vi "Lab Panel V5.31.vi"() -> ()   [LabVIEW 2017] (continued)
                n1120 = Equal?(x=w2128, y="RUN") -> (x = y?=w2130:bool)
                n1121 = And(x=w2130, y=w2131) -> (x .and. y?=w2129:bool)
                n1122 = case shown="True" w2129 {
                  tunnel: w2134 -> [_ w2139]
                  tunnel: w2133 -> [_ w2143]
                  frame False {
                  }
                  frame True {
                    n1123 = local read "SET LAB01-1"() -> (w2145:T6)
                    n1124 = local read "TDMS LAB01-1"() -> (w2138:refnum<k34>)
                    n1125 = Unbundle(w2145) -> ("CYCLES"=w2136:dbl, "T-RISE mins"=w2142:dbl)  [unwired: 3 out]
                    n1126 = case shown="\"CYCLE TEST\"" w2143 {
                      tunnel: w2142 -> [_ _ w2152]
                      tunnel: [w2147 w2149 w2152] -> w2141
                      tunnel: w2136 -> [w2147 w2149 _]
                      tunnel: ["CHART PASS" "CYCLE PASS" "T-RISE PASS"] -> w2140
                      frame "CHART TEST", Default {
                      }
                      frame "CYCLE TEST" {
                      }
                      frame "T-RISE TEST" {
                      }
                    }
                    n1127 = Unbundle(w2139) -> ("CYCLE"=w2144:dbl)  [unwired: 2 out]
                    n1128 = Increment(x=w2136) -> (x+1=w2137:dbl)
                    n1129 = Greater Or Equal?(x=w2144, y=w2137) -> (x >= y?=w2146:bool)
                    n1130 = case shown="True" w2146 {
                      tunnel: w2141 -> [w2156 _]
                      tunnel: w2140 -> [w2155 _]
                      tunnel: w2139 -> [w2154 _]
                      tunnel: w2138 -> [w2153 _]
                      frame True {
                        n1131 = stacked-sequence {
                          tunnel: w2156 -> [w2160 _]
                          tunnel: w2155 -> [w2158 w2164]
                          tunnel: w2154 -> [_ w2167]
                          tunnel: w2153 -> [w2157 _]
                          frame #0 {
                            n1132 = Build Array(w2158) -> (w2161:string[])
                            n1133 = Build Array(w2160) -> (w2159:dbl[])
                            n1134 = TDMS Write(0:w2157, 5:"TEST PASS", 7:w2161, 9:w2159) -> (15:w2163:errorcluster)  [unwired: 2 in, 3 out]
                            n1135 = local write "data file error"(w2163) -> ()
                          }
                          frame #1 {
                            n1136 = Bundle(cluster=w2167, "STATUS"=w2164) -> (w2165:T4)  [unwired: 2 in]
                            n1137 = local write "RESULT LAB01-1"(TRUE) -> ()
                            n1138 = local write "DISP LAB01-1"(w2165) -> ()
                          }
                        }
                      }
                      frame False {
                      }
                    }
                  }
                }
              }
              frame #1 {
                # "LAB01-2"
                n1139 = Less?(x=w2168, y=2) -> (x < y?=w2171:bool)
                n1140 = local read "DISP LAB01-2"() -> (w2173:T4)
                n1141 = Unbundle(w2173) -> ("STATUS"=w2174:string)  [unwired: 2 out]
                n1142 = Equal?(x=w2174, y="RUN") -> (x = y?=w2170:bool)
                n1143 = And(x=w2170, y=w2171) -> (x .and. y?=w2169:bool)
                n1144 = case shown="True" w2169 {
                  tunnel: w2173 -> [_ w2179]
                  tunnel: w2168 -> [_ w2183]
                  frame False {
                  }
                  frame True {
                    n1145 = local read "SET LAB01-2"() -> (w2185:T5)
                    n1146 = local read "TDMS LAB01-2"() -> (w2178:refnum<k34>)
                    n1147 = Unbundle(w2185) -> ("CYCLES"=w2176:dbl, "T-RISE mins"=w2182:dbl)  [unwired: 3 out]
                    n1148 = case shown="\"T-RISE TEST\"" w2183 {
                      tunnel: w2182 -> [_ _ w2192]
                      tunnel: [w2187 w2189 w2192] -> w2181
                      tunnel: w2176 -> [w2187 w2189 _]
                      tunnel: ["CHART PASS" "CYCLE PASS" "T-RISE PASS"] -> w2180
                      frame "CHART TEST", Default {
                      }
                      frame "CYCLE TEST" {
                      }
                      frame "T-RISE TEST" {
                      }
                    }
                    n1149 = Unbundle(w2179) -> ("CYCLE"=w2184:dbl)  [unwired: 2 out]
                    n1150 = Increment(x=w2176) -> (x+1=w2177:dbl)
                    n1151 = Greater Or Equal?(x=w2184, y=w2177) -> (x >= y?=w2186:bool)
                    n1152 = case shown="True" w2186 {
                      tunnel: w2181 -> [w2196 _]
                      tunnel: w2180 -> [w2195 _]
                      tunnel: w2179 -> [w2194 _]
                      tunnel: w2178 -> [w2193 _]
                      frame True {
                        n1153 = stacked-sequence {
                          tunnel: w2196 -> [w2200 _]
                          tunnel: w2195 -> [w2198 w2204]
                          tunnel: w2194 -> [_ w2207]
                          tunnel: w2193 -> [w2197 _]
                          frame #0 {
                            n1154 = Build Array(w2198) -> (w2201:string[])
                            n1155 = Build Array(w2200) -> (w2199:dbl[])
                            n1156 = TDMS Write(0:w2197, 5:"TEST PASS", 7:w2201, 9:w2199) -> (15:w2203:errorcluster)  [unwired: 2 in, 3 out]
                            n1157 = local write "data file error"(w2203) -> ()
                          }
                          frame #1 {
                            n1158 = Bundle(cluster=w2207, "STATUS"=w2204) -> (w2205:T4)  [unwired: 2 in]
                            n1159 = local write "RESULT LAB01-2"(TRUE) -> ()
                            n1160 = local write "DISP LAB01-2"(w2205) -> ()
                          }
                        }
                      }
                      frame False {
                      }
                    }
                  }
                }
              }
              frame #2 {
                # "LAB02-1"
                n1161 = Less?(x=w2208, y=2) -> (x < y?=w2211:bool)
                n1162 = local read "DISP LAB02-1"() -> (w2213:T4)
                n1163 = Unbundle(w2213) -> ("STATUS"=w2214:string)  [unwired: 2 out]
                n1164 = Equal?(x=w2214, y="RUN") -> (x = y?=w2210:bool)
                n1165 = And(x=w2210, y=w2211) -> (x .and. y?=w2209:bool)
                n1166 = case shown="True" w2209 {
                  tunnel: w2213 -> [_ w2219]
                  tunnel: w2208 -> [_ w2223]
                  frame False {
                  }
                  frame True {
                    n1167 = local read "TDMS LAB02-1"() -> (w2218:refnum<k34>)
                    n1168 = local read "SET LAB02-1"() -> (w2225:T5)
                    n1169 = Unbundle(w2219) -> ("CYCLE"=w2224:dbl)  [unwired: 2 out]
                    n1170 = Unbundle(w2225) -> ("CYCLES"=w2216:dbl, "T-RISE mins"=w2222:dbl)  [unwired: 3 out]
                    n1171 = case shown="\"T-RISE TEST\"" w2223 {
                      tunnel: w2222 -> [_ _ w2232]
                      tunnel: [w2227 w2229 w2232] -> w2221
                      tunnel: w2216 -> [w2227 w2229 _]
                      tunnel: ["CHART PASS" "CYCLE PASS" "T-RISE PASS"] -> w2220
                      frame "CHART TEST", Default {
                      }
                      frame "CYCLE TEST" {
                      }
                      frame "T-RISE TEST" {
                      }
                    }
                    n1172 = Increment(x=w2216) -> (x+1=w2217:dbl)
                    n1173 = Greater Or Equal?(x=w2224, y=w2217) -> (x >= y?=w2226:bool)
                    n1174 = case shown="True" w2226 {
                      tunnel: w2221 -> [w2236 _]
                      tunnel: w2220 -> [w2235 _]
                      tunnel: w2219 -> [w2234 _]
                      tunnel: w2218 -> [w2233 _]
                      frame True {
                        n1175 = stacked-sequence {
                          tunnel: w2236 -> [w2240 _]
                          tunnel: w2235 -> [w2238 w2244]
                          tunnel: w2234 -> [_ w2247]
                          tunnel: w2233 -> [w2237 _]
                          frame #0 {
                            n1176 = Build Array(w2238) -> (w2241:string[])
                            n1177 = Build Array(w2240) -> (w2239:dbl[])
                            n1178 = TDMS Write(0:w2237, 5:"TEST PASS", 7:w2241, 9:w2239) -> (15:w2243:errorcluster)  [unwired: 2 in, 3 out]
                            n1179 = local write "data file error"(w2243) -> ()
                          }
                          frame #1 {
                            n1180 = Bundle(cluster=w2247, "STATUS"=w2244) -> (w2245:T4)  [unwired: 2 in]
                            n1181 = local write "RESULT LAB02-1"(TRUE) -> ()
                            n1182 = local write "DISP LAB02-1"(w2245) -> ()
                          }
                        }
                      }
                      frame False {
                      }
                    }
                  }
                }
              }
              frame #3 {
                # "LAB02-2"
                n1183 = Less?(x=w2248, y=2) -> (x < y?=w2251:bool)
                n1184 = local read "DISP LAB02-2"() -> (w2253:T4)
                n1185 = Unbundle(w2253) -> ("STATUS"=w2254:string)  [unwired: 2 out]
                n1186 = Equal?(x=w2254, y="RUN") -> (x = y?=w2250:bool)
                n1187 = And(x=w2250, y=w2251) -> (x .and. y?=w2249:bool)
                n1188 = case shown="True" w2249 {
                  tunnel: w2253 -> [_ w2259]
                  tunnel: w2248 -> [_ w2263]
                  frame False {
                  }
                  frame True {
                    n1189 = local read "TDMS LAB02-2"() -> (w2258:refnum<k34>)
                    n1190 = local read "SET LAB02-2"() -> (w2265:T5)
                    n1191 = Unbundle(w2259) -> ("CYCLE"=w2264:dbl)  [unwired: 2 out]
                    n1192 = Unbundle(w2265) -> ("CYCLES"=w2256:dbl, "T-RISE mins"=w2262:dbl)  [unwired: 3 out]
                    n1193 = case shown="\"T-RISE TEST\"" w2263 {
                      tunnel: w2262 -> [_ _ w2272]
                      tunnel: [w2267 w2269 w2272] -> w2261
                      tunnel: w2256 -> [w2267 w2269 _]
                      tunnel: ["CHART PASS" "CYCLE PASS" "T-RISE PASS"] -> w2260
                      frame "CHART TEST", Default {
                      }
                      frame "CYCLE TEST" {
                      }
                      frame "T-RISE TEST" {
                      }
                    }
                    n1194 = Increment(x=w2256) -> (x+1=w2257:dbl)
                    n1195 = Greater Or Equal?(x=w2264, y=w2257) -> (x >= y?=w2266:bool)
                    n1196 = case shown="True" w2266 {
                      tunnel: w2261 -> [w2276 _]
                      tunnel: w2260 -> [w2275 _]
                      tunnel: w2259 -> [w2274 _]
                      tunnel: w2258 -> [w2273 _]
                      frame True {
                        n1197 = stacked-sequence {
                          tunnel: w2276 -> [w2280 _]
                          tunnel: w2275 -> [w2278 w2284]
                          tunnel: w2274 -> [_ w2287]
                          tunnel: w2273 -> [w2277 _]
                          frame #0 {
                            n1198 = Build Array(w2278) -> (w2281:string[])
                            n1199 = Build Array(w2280) -> (w2279:dbl[])
                            n1200 = TDMS Write(0:w2277, 5:"TEST PASS", 7:w2281, 9:w2279) -> (15:w2283:errorcluster)  [unwired: 2 in, 3 out]
                            n1201 = local write "data file error"(w2283) -> ()
                          }
                          frame #1 {
                            n1202 = Bundle(cluster=w2287, "STATUS"=w2284) -> (w2285:T4)  [unwired: 2 in]
                            n1203 = local write "RESULT LAB02-2"(TRUE) -> ()
                            n1204 = local write "DISP LAB02-2"(w2285) -> ()
                          }
                        }
                      }
                      frame False {
                      }
                    }
                  }
                }
              }
              frame #4 {
                # "LAB03-1"
                n1205 = Less?(x=w2288, y=2) -> (x < y?=w2291:bool)
                n1206 = local read "DISP LAB03-1"() -> (w2293:T4)
                n1207 = Unbundle(w2293) -> ("STATUS"=w2294:string)  [unwired: 2 out]
                n1208 = Equal?(x=w2294, y="RUN") -> (x = y?=w2290:bool)
                n1209 = And(x=w2290, y=w2291) -> (x .and. y?=w2289:bool)
                n1210 = case shown="True" w2289 {
                  tunnel: w2293 -> [_ w2299]
                  tunnel: w2288 -> [_ w2303]
                  frame False {
                  }
                  frame True {
                    n1211 = local read "TDMS LAB03-1"() -> (w2298:refnum<k34>)
                    n1212 = local read "SET LAB03-1"() -> (w2305:T5)
                    n1213 = Unbundle(w2299) -> ("CYCLE"=w2304:dbl)  [unwired: 2 out]
                    n1214 = Unbundle(w2305) -> ("CYCLES"=w2296:dbl, "T-RISE mins"=w2302:dbl)  [unwired: 3 out]
                    n1215 = case shown="\"T-RISE TEST\"" w2303 {
                      tunnel: w2302 -> [_ _ w2312]
                      tunnel: [w2307 w2309 w2312] -> w2301
                      tunnel: w2296 -> [w2307 w2309 _]
                      tunnel: ["CHART PASS" "CYCLE PASS" "T-RISE PASS"] -> w2300
                      frame "CHART TEST", Default {
                      }
                      frame "CYCLE TEST" {
                      }
                      frame "T-RISE TEST" {
                      }
                    }
                    n1216 = Increment(x=w2296) -> (x+1=w2297:dbl)
                    n1217 = Greater Or Equal?(x=w2304, y=w2297) -> (x >= y?=w2306:bool)
                    n1218 = case shown="True" w2306 {
                      tunnel: w2301 -> [w2316 _]
                      tunnel: w2300 -> [w2315 _]
                      tunnel: w2299 -> [w2314 _]
                      tunnel: w2298 -> [w2313 _]
                      frame True {
                        n1219 = stacked-sequence {
                          tunnel: w2316 -> [w2320 _]
                          tunnel: w2315 -> [w2318 w2324]
                          tunnel: w2314 -> [_ w2327]
                          tunnel: w2313 -> [w2317 _]
                          frame #0 {
                            n1220 = Build Array(w2318) -> (w2321:string[])
                            n1221 = Build Array(w2320) -> (w2319:dbl[])
                            n1222 = TDMS Write(0:w2317, 5:"TEST PASS", 7:w2321, 9:w2319) -> (15:w2323:errorcluster)  [unwired: 2 in, 3 out]
                            n1223 = local write "data file error"(w2323) -> ()
                          }
                          frame #1 {
                            n1224 = Bundle(cluster=w2327, "STATUS"=w2324) -> (w2325:T4)  [unwired: 2 in]
                            n1225 = local write "RESULT LAB03-1"(TRUE) -> ()
                            n1226 = local write "DISP LAB03-1"(w2325) -> ()
                          }
                        }
                      }
                      frame False {
                      }
                    }
                  }
                }
              }
              frame #5 {
                # "LAB03-2"
                n1227 = Less?(x=w2328, y=2) -> (x < y?=w2331:bool)
                n1228 = local read "DISP LAB03-2"() -> (w2333:T4)
                n1229 = Unbundle(w2333) -> ("STATUS"=w2334:string)  [unwired: 2 out]
                n1230 = Equal?(x=w2334, y="RUN") -> (x = y?=w2330:bool)
                n1231 = And(x=w2330, y=w2331) -> (x .and. y?=w2329:bool)
                n1232 = case shown="True" w2329 {
                  tunnel: w2333 -> [_ w2339]
                  tunnel: w2328 -> [_ w2343]
                  frame False {
                  }
                  frame True {
                    n1233 = local read "TDMS LAB03-2"() -> (w2338:refnum<k34>)
                    n1234 = local read "SET LAB03-2"() -> (w2345:T5)
                    n1235 = Unbundle(w2339) -> ("CYCLE"=w2344:dbl)  [unwired: 2 out]
                    n1236 = Unbundle(w2345) -> ("CYCLES"=w2336:dbl, "T-RISE mins"=w2342:dbl)  [unwired: 3 out]
                    n1237 = case shown="\"T-RISE TEST\"" w2343 {
                      tunnel: w2342 -> [_ _ w2352]
                      tunnel: [w2347 w2349 w2352] -> w2341
                      tunnel: w2336 -> [w2347 w2349 _]
                      tunnel: ["CHART PASS" "CYCLE PASS" "T-RISE PASS"] -> w2340
                      frame "CHART TEST", Default {
                      }
                      frame "CYCLE TEST" {
                      }
                      frame "T-RISE TEST" {
                      }
                    }
                    n1238 = Increment(x=w2336) -> (x+1=w2337:dbl)
                    n1239 = Greater Or Equal?(x=w2344, y=w2337) -> (x >= y?=w2346:bool)
                    n1240 = case shown="True" w2346 {
                      tunnel: w2341 -> [w2356 _]
                      tunnel: w2340 -> [w2355 _]
                      tunnel: w2339 -> [w2354 _]
                      tunnel: w2338 -> [w2353 _]
                      frame True {
                        n1241 = stacked-sequence {
                          tunnel: w2356 -> [w2360 _]
                          tunnel: w2355 -> [w2358 w2364]
                          tunnel: w2354 -> [_ w2367]
                          tunnel: w2353 -> [w2357 _]
                          frame #0 {
                            n1242 = Build Array(w2358) -> (w2361:string[])
                            n1243 = Build Array(w2360) -> (w2359:dbl[])
                            n1244 = TDMS Write(0:w2357, 5:"TEST PASS", 7:w2361, 9:w2359) -> (15:w2363:errorcluster)  [unwired: 2 in, 3 out]
                            n1245 = local write "data file error"(w2363) -> ()
                          }
                          frame #1 {
                            n1246 = Bundle(cluster=w2367, "STATUS"=w2364) -> (w2365:T4)  [unwired: 2 in]
                            n1247 = local write "RESULT LAB03-2"(TRUE) -> ()
                            n1248 = local write "DISP LAB03-2"(w2365) -> ()
                          }
                        }
                      }
                      frame False {
                      }
                    }
                  }
                }
              }
              frame #6 {
                # "LAB04-1"
                n1249 = Less?(x=w2368, y=2) -> (x < y?=w2371:bool)
                n1250 = local read "DISP LAB04-1"() -> (w2373:T4)
                n1251 = Unbundle(w2373) -> ("STATUS"=w2374:string)  [unwired: 2 out]
                n1252 = Equal?(x=w2374, y="RUN") -> (x = y?=w2370:bool)
                n1253 = And(x=w2370, y=w2371) -> (x .and. y?=w2369:bool)
                n1254 = case shown="True" w2369 {
                  tunnel: w2373 -> [_ w2379]
                  tunnel: w2368 -> [_ w2383]
                  frame False {
                  }
                  frame True {
                    n1255 = local read "TDMS LAB04-1"() -> (w2378:refnum<k34>)
                    n1256 = local read "SET LAB04-1"() -> (w2385:T5)
                    n1257 = Unbundle(w2379) -> ("CYCLE"=w2384:dbl)  [unwired: 2 out]
                    n1258 = Unbundle(w2385) -> ("CYCLES"=w2376:dbl, "T-RISE mins"=w2382:dbl)  [unwired: 3 out]
                    n1259 = case shown="\"T-RISE TEST\"" w2383 {
                      tunnel: w2382 -> [_ _ w2392]
                      tunnel: [w2387 w2389 w2392] -> w2381
                      tunnel: w2376 -> [w2387 w2389 _]
                      tunnel: ["CHART PASS" "CYCLE PASS" "T-RISE PASS"] -> w2380
                      frame "CHART TEST", Default {
                      }
                      frame "CYCLE TEST" {
                      }
                      frame "T-RISE TEST" {
                      }
                    }
                    n1260 = Increment(x=w2376) -> (x+1=w2377:dbl)
                    n1261 = Greater Or Equal?(x=w2384, y=w2377) -> (x >= y?=w2386:bool)
                    n1262 = case shown="True" w2386 {
                      tunnel: w2381 -> [w2396 _]
                      tunnel: w2380 -> [w2395 _]
                      tunnel: w2379 -> [w2394 _]
                      tunnel: w2378 -> [w2393 _]
                      frame True {
                        n1263 = stacked-sequence {
                          tunnel: w2396 -> [w2400 _]
                          tunnel: w2395 -> [w2398 w2404]
                          tunnel: w2394 -> [_ w2407]
                          tunnel: w2393 -> [w2397 _]
                          frame #0 {
                            n1264 = Build Array(w2398) -> (w2401:string[])
                            n1265 = Build Array(w2400) -> (w2399:dbl[])
                            n1266 = TDMS Write(0:w2397, 5:"TEST PASS", 7:w2401, 9:w2399) -> (15:w2403:errorcluster)  [unwired: 2 in, 3 out]
                            n1267 = local write "data file error"(w2403) -> ()
                          }
                          frame #1 {
                            n1268 = Bundle(cluster=w2407, "STATUS"=w2404) -> (w2405:T4)  [unwired: 2 in]
                            n1269 = local write "RESULT LAB04-1"(TRUE) -> ()
                            n1270 = local write "DISP LAB04-1"(w2405) -> ()
                          }
                        }
                      }
                      frame False {
                      }
                    }
                  }
                }
              }
              frame #7 {
                # "LAB04-2"
                n1271 = Less?(x=w2408, y=2) -> (x < y?=w2411:bool)
                n1272 = local read "DISP LAB04-2"() -> (w2413:T4)
                n1273 = Unbundle(w2413) -> ("STATUS"=w2414:string)  [unwired: 2 out]
                n1274 = Equal?(x=w2414, y="RUN") -> (x = y?=w2410:bool)
                n1275 = And(x=w2410, y=w2411) -> (x .and. y?=w2409:bool)
                n1276 = case shown="True" w2409 {
                  tunnel: w2413 -> [_ w2419]
                  tunnel: w2408 -> [_ w2423]
                  frame False {
                  }
                  frame True {
                    n1277 = local read "TDMS LAB04-2"() -> (w2418:refnum<k34>)
                    n1278 = local read "SET LAB04-2"() -> (w2425:T5)
                    n1279 = Unbundle(w2419) -> ("CYCLE"=w2424:dbl)  [unwired: 2 out]
                    n1280 = Unbundle(w2425) -> ("CYCLES"=w2416:dbl, "T-RISE mins"=w2422:dbl)  [unwired: 3 out]
                    n1281 = case shown="\"T-RISE TEST\"" w2423 {
                      tunnel: w2422 -> [_ _ w2432]
                      tunnel: [w2427 w2429 w2432] -> w2421
                      tunnel: w2416 -> [w2427 w2429 _]
                      tunnel: ["CHART PASS" "CYCLE PASS" "T-RISE PASS"] -> w2420
                      frame "CHART TEST", Default {
                      }
                      frame "CYCLE TEST" {
                      }
                      frame "T-RISE TEST" {
                      }
                    }
                    n1282 = Increment(x=w2416) -> (x+1=w2417:dbl)
                    n1283 = Greater Or Equal?(x=w2424, y=w2417) -> (x >= y?=w2426:bool)
                    n1284 = case shown="True" w2426 {
                      tunnel: w2421 -> [w2436 _]
                      tunnel: w2420 -> [w2435 _]
                      tunnel: w2419 -> [w2434 _]
                      tunnel: w2418 -> [w2433 _]
                      frame True {
                        n1285 = stacked-sequence {
                          tunnel: w2436 -> [w2440 _]
                          tunnel: w2435 -> [w2438 w2444]
                          tunnel: w2434 -> [_ w2447]
                          tunnel: w2433 -> [w2437 _]
                          frame #0 {
                            n1286 = Build Array(w2438) -> (w2441:string[])
                            n1287 = Build Array(w2440) -> (w2439:dbl[])
                            n1288 = TDMS Write(0:w2437, 5:"TEST PASS", 7:w2441, 9:w2439) -> (15:w2443:errorcluster)  [unwired: 2 in, 3 out]
                            n1289 = local write "data file error"(w2443) -> ()
                          }
                          frame #1 {
                            n1290 = Bundle(cluster=w2447, "STATUS"=w2444) -> (w2445:T4)  [unwired: 2 in]
                            n1291 = local write "RESULT LAB04-2"(TRUE) -> ()
                            n1292 = local write "DISP LAB04-2"(w2445) -> ()
                          }
                        }
                      }
                      frame False {
                      }
                    }
                  }
                }
              }
              frame #8 {
                # "LAB05-1"
                n1293 = Less?(x=w2448, y=2) -> (x < y?=w2451:bool)
                n1294 = local read "DISP LAB05-1"() -> (w2453:T4)
                n1295 = Unbundle(w2453) -> ("STATUS"=w2454:string)  [unwired: 2 out]
                n1296 = Equal?(x=w2454, y="RUN") -> (x = y?=w2450:bool)
                n1297 = And(x=w2450, y=w2451) -> (x .and. y?=w2449:bool)
                n1298 = case shown="True" w2449 {
                  tunnel: w2453 -> [_ w2459]
                  tunnel: w2448 -> [_ w2463]
                  frame False {
                  }
                  frame True {
                    n1299 = local read "TDMS LAB05-1"() -> (w2458:refnum<k34>)
                    n1300 = local read "SET LAB05-1"() -> (w2465:T5)
                    n1301 = Unbundle(w2459) -> ("CYCLE"=w2464:dbl)  [unwired: 2 out]
                    n1302 = Unbundle(w2465) -> ("CYCLES"=w2456:dbl, "T-RISE mins"=w2462:dbl)  [unwired: 3 out]
                    n1303 = case shown="\"T-RISE TEST\"" w2463 {
                      tunnel: w2462 -> [_ _ w2472]
                      tunnel: [w2467 w2469 w2472] -> w2461
                      tunnel: w2456 -> [w2467 w2469 _]
                      tunnel: ["CHART PASS" "CYCLE PASS" "T-RISE PASS"] -> w2460
                      frame "CHART TEST", Default {
                      }
                      frame "CYCLE TEST" {
                      }
                      frame "T-RISE TEST" {
                      }
                    }
                    n1304 = Increment(x=w2456) -> (x+1=w2457:dbl)
                    n1305 = Greater Or Equal?(x=w2464, y=w2457) -> (x >= y?=w2466:bool)
                    n1306 = case shown="True" w2466 {
                      tunnel: w2461 -> [w2476 _]
                      tunnel: w2460 -> [w2475 _]
                      tunnel: w2459 -> [w2474 _]
                      tunnel: w2458 -> [w2473 _]
                      frame True {
                        n1307 = stacked-sequence {
                          tunnel: w2476 -> [w2480 _]
                          tunnel: w2475 -> [w2478 w2484]
                          tunnel: w2474 -> [_ w2487]
                          tunnel: w2473 -> [w2477 _]
                          frame #0 {
                            n1308 = Build Array(w2478) -> (w2481:string[])
                            n1309 = Build Array(w2480) -> (w2479:dbl[])
                            n1310 = TDMS Write(0:w2477, 5:"TEST PASS", 7:w2481, 9:w2479) -> (15:w2483:errorcluster)  [unwired: 2 in, 3 out]
                            n1311 = local write "data file error"(w2483) -> ()
                          }
                          frame #1 {
                            n1312 = Bundle(cluster=w2487, "STATUS"=w2484) -> (w2485:T4)  [unwired: 2 in]
                            n1313 = local write "RESULT LAB05-1"(TRUE) -> ()
                            n1314 = local write "DISP LAB05-1"(w2485) -> ()
                          }
                        }
                      }
                      frame False {
                      }
                    }
                  }
                }
              }
              frame #9 {
                # "LAB05-2"
                n1315 = Less?(x=w2488, y=2) -> (x < y?=w2491:bool)
                n1316 = local read "DISP LAB05-2"() -> (w2493:T4)
                n1317 = Unbundle(w2493) -> ("STATUS"=w2494:string)  [unwired: 2 out]
                n1318 = Equal?(x=w2494, y="RUN") -> (x = y?=w2490:bool)
                n1319 = And(x=w2490, y=w2491) -> (x .and. y?=w2489:bool)
                n1320 = case shown="True" w2489 {
                  tunnel: w2493 -> [_ w2499]
                  tunnel: w2488 -> [_ w2503]
                  frame False {
                  }
                  frame True {
                    n1321 = local read "TDMS LAB05-2"() -> (w2498:refnum<k34>)
                    n1322 = local read "SET LAB05-2"() -> (w2505:T5)
                    n1323 = Unbundle(w2499) -> ("CYCLE"=w2504:dbl)  [unwired: 2 out]
                    n1324 = Unbundle(w2505) -> ("CYCLES"=w2496:dbl, "T-RISE mins"=w2502:dbl)  [unwired: 3 out]
                    n1325 = case shown="\"T-RISE TEST\"" w2503 {
                      tunnel: w2502 -> [_ _ w2512]
                      tunnel: [w2507 w2509 w2512] -> w2501
                      tunnel: w2496 -> [w2507 w2509 _]
                      tunnel: ["CHART PASS" "CYCLE PASS" "T-RISE PASS"] -> w2500
                      frame "CHART TEST", Default {
                      }
                      frame "CYCLE TEST" {
                      }
                      frame "T-RISE TEST" {
                      }
                    }
                    n1326 = Increment(x=w2496) -> (x+1=w2497:dbl)
                    n1327 = Greater Or Equal?(x=w2504, y=w2497) -> (x >= y?=w2506:bool)
                    n1328 = case shown="True" w2506 {
                      tunnel: w2501 -> [w2516 _]
                      tunnel: w2500 -> [w2515 _]
                      tunnel: w2499 -> [w2514 _]
                      tunnel: w2498 -> [w2513 _]
                      frame True {
                        n1329 = stacked-sequence {
                          tunnel: w2516 -> [w2520 _]
                          tunnel: w2515 -> [w2518 w2524]
                          tunnel: w2514 -> [_ w2527]
                          tunnel: w2513 -> [w2517 _]
                          frame #0 {
                            n1330 = Build Array(w2518) -> (w2521:string[])
                            n1331 = Build Array(w2520) -> (w2519:dbl[])
                            n1332 = TDMS Write(0:w2517, 5:"TEST PASS", 7:w2521, 9:w2519) -> (15:w2523:errorcluster)  [unwired: 2 in, 3 out]
                            n1333 = local write "data file error"(w2523) -> ()
                          }
                          frame #1 {
                            n1334 = Bundle(cluster=w2527, "STATUS"=w2524) -> (w2525:T4)  [unwired: 2 in]
                            n1335 = local write "RESULT LAB05-2"(TRUE) -> ()
                            n1336 = local write "DISP LAB05-2"(w2525) -> ()
                          }
                        }
                      }
                      frame False {
                      }
                    }
                  }
                }
              }
            }
          }
          frame #6 {
            # "check if test cycles reached for temperature rise test"
            n1337 = stacked-sequence {
              tunnel: w2557 -> [_ _ _ _ _ _ _ _ _ _]
              tunnel: w2556 -> [_ _ _ _ _ _ _ _ _ _]
              tunnel: w2555 -> [_ _ _ _ _ _ _ _ _ _]
              tunnel: w2554 -> [_ _ _ _ _ _ _ _ _ _]
              tunnel: w2553 -> [_ _ _ _ _ _ _ _ _ _]
              tunnel: w2552 -> [_ _ _ _ _ _ _ _ _ _]
              tunnel: w2551 -> [_ _ _ _ _ _ _ _ _ _]
              tunnel: w2550 -> [_ _ _ _ _ _ _ _ _ _]
              tunnel: w2549 -> [_ _ _ _ _ _ _ _ _ _]
              tunnel: w2548 -> [_ _ _ _ _ _ _ _ _ _]
              tunnel: w2547 -> [w2563 _ _ _ _ _ _ _ _ _]
              tunnel: w2537 -> [w2558 _ _ _ _ _ _ _ _ _]
              tunnel: w2546 -> [_ w2589 _ _ _ _ _ _ _ _]
              tunnel: w2545 -> [_ _ w2619 _ _ _ _ _ _ _]
              tunnel: w2544 -> [_ _ _ w2649 _ _ _ _ _ _]
              tunnel: w2543 -> [_ _ _ _ w2679 _ _ _ _ _]
              tunnel: w2542 -> [_ _ _ _ _ w2709 _ _ _ _]
              tunnel: w2541 -> [_ _ _ _ _ _ w2739 _ _ _]
              tunnel: w2540 -> [_ _ _ _ _ _ _ w2769 _ _]
              tunnel: w2539 -> [_ _ _ _ _ _ _ _ w2799 _]
              tunnel: w2538 -> [_ _ _ _ _ _ _ _ _ w2829]
              tunnel: w2536 -> [_ w2588 _ _ _ _ _ _ _ _]
              tunnel: w2535 -> [_ _ w2618 _ _ _ _ _ _ _]
              tunnel: w2534 -> [_ _ _ w2648 _ _ _ _ _ _]
              tunnel: w2533 -> [_ _ _ _ w2678 _ _ _ _ _]
              tunnel: w2532 -> [_ _ _ _ _ w2708 _ _ _ _]
              tunnel: w2531 -> [_ _ _ _ _ _ w2738 _ _ _]
              tunnel: w2530 -> [_ _ _ _ _ _ _ w2768 _ _]
              tunnel: w2529 -> [_ _ _ _ _ _ _ _ w2798 _]
              tunnel: w2528 -> [_ _ _ _ _ _ _ _ _ w2828]
              frame #0 {
                # "LAB01-1"
                n1338 = Equal?(x=w2563, y=2) -> (x = y?=w2561:bool)
                n1339 = local read "DISP LAB01-1"() -> (w2564:T4)
                n1340 = Unbundle By Name(w2564) -> ("STATUS"=w2565:string)
                n1341 = Equal?(x=w2565, y="RUN") -> (x = y?=w2560:bool)
                n1342 = And(x=w2560, y=w2561) -> (x .and. y?=w2559:bool)
                n1343 = case shown="True" w2559 {
                  tunnel: w2564 -> [_ w2568]
                  tunnel: w2558 -> [_ w2571]
                  frame False {
                  }
                  frame True {
                    n1344 = Unbundle By Name(w2568) -> ("CYCLE"=w2572:dbl)
                    n1345 = local read "SET LAB01-1"() -> (w2570:T6)
                    n1346 = local read "TDMS LAB01-1"() -> (w2567:refnum<k34>)
                    n1347 = Unbundle(w2570) -> ("T-RISE mins"=w2569:dbl)  [unwired: 4 out]
                    n1348 = Greater Or Equal?(x=w2572, y=w2571) -> (x >= y?=w2573:bool)
                    n1349 = case shown="True" w2573 {
                      tunnel: w2569 -> [w2576 _]
                      tunnel: w2568 -> [w2575 _]
                      tunnel: w2567 -> [w2574 _]
                      frame True {
                        n1350 = stacked-sequence {
                          tunnel: w2576 -> [w2579 _]
                          tunnel: w2575 -> [_ w2584]
                          tunnel: w2574 -> [w2577 _]
                          frame #0 {
                            n1351 = Build Array("T-RISE") -> (w2581:string[])
                            n1352 = Build Array(w2579) -> (w2580:dbl[])
                            n1353 = TDMS Write(0:w2577, 5:"TEST PASS", 7:w2581, 9:w2580) -> (15:w2583:errorcluster)  [unwired: 2 in, 3 out]
                            n1354 = local write "data file error"(w2583) -> ()
                          }
                          frame #1 {
                            n1355 = Bundle(cluster=w2584, "STATUS"="T-RISE PASS") -> (w2586:T4)  [unwired: 2 in]
                            n1356 = local write "RESULT LAB01-1"(TRUE) -> ()
                            n1357 = local write "DISP LAB01-1"(w2586) -> ()
                          }
                        }
                      }
                      frame False {
                      }
                    }
                  }
                }
              }
              frame #1 {
                # "LAB01-2"
                n1358 = Equal?(x=w2589, y=2) -> (x = y?=w2592:bool)
                n1359 = local read "DISP LAB01-2"() -> (w2594:T4)
                n1360 = Unbundle(w2594) -> ("STATUS"=w2595:string)  [unwired: 2 out]
                n1361 = Equal?(x=w2595, y="RUN") -> (x = y?=w2591:bool)
                n1362 = And(x=w2591, y=w2592) -> (x .and. y?=w2590:bool)
                n1363 = case shown="True" w2590 {
                  tunnel: w2594 -> [_ w2598]
                  tunnel: w2588 -> [_ w2601]
                  frame False {
                  }
                  frame True {
                    n1364 = local read "SET LAB01-2"() -> (w2600:T5)
                    n1365 = local read "TDMS LAB01-2"() -> (w2597:refnum<k34>)
                    n1366 = Unbundle(w2598) -> ("CYCLE"=w2602:dbl)  [unwired: 2 out]
                    n1367 = Unbundle(w2600) -> ("T-RISE mins"=w2599:dbl)  [unwired: 4 out]
                    n1368 = Greater Or Equal?(x=w2602, y=w2601) -> (x >= y?=w2603:bool)
                    n1369 = case shown="True" w2603 {
                      tunnel: w2599 -> [w2606 _]
                      tunnel: w2598 -> [w2605 _]
                      tunnel: w2597 -> [w2604 _]
                      frame True {
                        n1370 = stacked-sequence {
                          tunnel: w2606 -> [w2609 _]
                          tunnel: w2605 -> [_ w2614]
                          tunnel: w2604 -> [w2607 _]
                          frame #0 {
                            n1371 = Build Array("T-RISE") -> (w2611:string[])
                            n1372 = Build Array(w2609) -> (w2610:dbl[])
                            n1373 = TDMS Write(0:w2607, 5:"TEST PASS", 7:w2611, 9:w2610) -> (15:w2613:errorcluster)  [unwired: 2 in, 3 out]
                            n1374 = local write "data file error"(w2613) -> ()
                          }
                          frame #1 {
                            n1375 = Bundle(cluster=w2614, "STATUS"="T-RISE PASS") -> (w2616:T4)  [unwired: 2 in]
                            n1376 = local write "RESULT LAB01-2"(TRUE) -> ()
                            n1377 = local write "DISP LAB01-2"(w2616) -> ()
                          }
                        }
                      }
                      frame False {
                      }
                    }
                  }
                }
              }
              frame #2 {
                # "LAB02-1"
                n1378 = Equal?(x=w2619, y=2) -> (x = y?=w2622:bool)
                n1379 = local read "DISP LAB02-1"() -> (w2624:T4)
                n1380 = Unbundle(w2624) -> ("STATUS"=w2625:string)  [unwired: 2 out]
                n1381 = Equal?(x=w2625, y="RUN") -> (x = y?=w2621:bool)
                n1382 = And(x=w2621, y=w2622) -> (x .and. y?=w2620:bool)
                n1383 = case shown="True" w2620 {
                  tunnel: w2624 -> [_ w2628]
                  tunnel: w2618 -> [_ w2631]
                  frame False {
                  }
                  frame True {
                    n1384 = local read "SET LAB02-1"() -> (w2630:T5)
                    n1385 = local read "TDMS LAB02-1"() -> (w2627:refnum<k34>)
                    n1386 = Unbundle(w2628) -> ("CYCLE"=w2632:dbl)  [unwired: 2 out]
                    n1387 = Unbundle(w2630) -> ("T-RISE mins"=w2629:dbl)  [unwired: 4 out]
                    n1388 = Greater Or Equal?(x=w2632, y=w2631) -> (x >= y?=w2633:bool)
                    n1389 = case shown="True" w2633 {
                      tunnel: w2629 -> [w2636 _]
                      tunnel: w2628 -> [w2635 _]
                      tunnel: w2627 -> [w2634 _]
                      frame True {
                        n1390 = stacked-sequence {
                          tunnel: w2636 -> [w2639 _]
                          tunnel: w2635 -> [_ w2644]
                          tunnel: w2634 -> [w2637 _]
                          frame #0 {
                            n1391 = Build Array("T-RISE") -> (w2641:string[])
                            n1392 = Build Array(w2639) -> (w2640:dbl[])
                            n1393 = TDMS Write(0:w2637, 5:"TEST PASS", 7:w2641, 9:w2640) -> (15:w2643:errorcluster)  [unwired: 2 in, 3 out]
                            n1394 = local write "data file error"(w2643) -> ()
                          }
                          frame #1 {
                            n1395 = Bundle(cluster=w2644, "STATUS"="T-RISE PASS") -> (w2646:T4)  [unwired: 2 in]
                            n1396 = local write "RESULT LAB02-1"(TRUE) -> ()
                            n1397 = local write "DISP LAB02-1"(w2646) -> ()
                          }
                        }
                      }
                      frame False {
                      }
                    }
                  }
                }
              }
              frame #3 {
                # "LAB02-2"
                n1398 = Equal?(x=w2649, y=2) -> (x = y?=w2652:bool)
                n1399 = local read "DISP LAB02-2"() -> (w2654:T4)
                n1400 = Unbundle(w2654) -> ("STATUS"=w2655:string)  [unwired: 2 out]
                n1401 = Equal?(x=w2655, y="RUN") -> (x = y?=w2651:bool)
                n1402 = And(x=w2651, y=w2652) -> (x .and. y?=w2650:bool)
                n1403 = case shown="True" w2650 {
                  tunnel: w2654 -> [_ w2658]
                  tunnel: w2648 -> [_ w2661]
                  frame False {
                  }
                  frame True {
                    n1404 = local read "SET LAB02-2"() -> (w2660:T5)
                    n1405 = local read "TDMS LAB02-2"() -> (w2657:refnum<k34>)
                    n1406 = Unbundle(w2658) -> ("CYCLE"=w2662:dbl)  [unwired: 2 out]
                    n1407 = Unbundle(w2660) -> ("T-RISE mins"=w2659:dbl)  [unwired: 4 out]
                    n1408 = Greater Or Equal?(x=w2662, y=w2661) -> (x >= y?=w2663:bool)
                    n1409 = case shown="True" w2663 {
                      tunnel: w2659 -> [w2666 _]
                      tunnel: w2658 -> [w2665 _]
                      tunnel: w2657 -> [w2664 _]
                      frame True {
                        n1410 = stacked-sequence {
                          tunnel: w2666 -> [w2669 _]
                          tunnel: w2665 -> [_ w2674]
                          tunnel: w2664 -> [w2667 _]
                          frame #0 {
                            n1411 = Build Array("T-RISE") -> (w2671:string[])
                            n1412 = Build Array(w2669) -> (w2670:dbl[])
                            n1413 = TDMS Write(0:w2667, 5:"TEST PASS", 7:w2671, 9:w2670) -> (15:w2673:errorcluster)  [unwired: 2 in, 3 out]
                            n1414 = local write "data file error"(w2673) -> ()
                          }
                          frame #1 {
                            n1415 = Bundle(cluster=w2674, "STATUS"="T-RISE PASS") -> (w2676:T4)  [unwired: 2 in]
                            n1416 = local write "RESULT LAB02-2"(TRUE) -> ()
                            n1417 = local write "DISP LAB02-2"(w2676) -> ()
                          }
                        }
                      }
                      frame False {
                      }
                    }
                  }
                }
              }
              frame #4 {
                # "LAB03-1"
                n1418 = Equal?(x=w2679, y=2) -> (x = y?=w2682:bool)
                n1419 = local read "DISP LAB03-1"() -> (w2684:T4)
                n1420 = Unbundle(w2684) -> ("STATUS"=w2685:string)  [unwired: 2 out]
                n1421 = Equal?(x=w2685, y="RUN") -> (x = y?=w2681:bool)
                n1422 = And(x=w2681, y=w2682) -> (x .and. y?=w2680:bool)
                n1423 = case shown="True" w2680 {
                  tunnel: w2684 -> [_ w2688]
                  tunnel: w2678 -> [_ w2691]
                  frame False {
                  }
                  frame True {
                    n1424 = local read "SET LAB03-1"() -> (w2690:T5)
                    n1425 = local read "TDMS LAB03-1"() -> (w2687:refnum<k34>)
                    n1426 = Unbundle(w2688) -> ("CYCLE"=w2692:dbl)  [unwired: 2 out]
                    n1427 = Unbundle(w2690) -> ("T-RISE mins"=w2689:dbl)  [unwired: 4 out]
                    n1428 = Greater Or Equal?(x=w2692, y=w2691) -> (x >= y?=w2693:bool)
                    n1429 = case shown="True" w2693 {
                      tunnel: w2689 -> [w2696 _]
                      tunnel: w2688 -> [w2695 _]
                      tunnel: w2687 -> [w2694 _]
                      frame True {
                        n1430 = stacked-sequence {
                          tunnel: w2696 -> [w2699 _]
                          tunnel: w2695 -> [_ w2704]
                          tunnel: w2694 -> [w2697 _]
                          frame #0 {
                            n1431 = Build Array("T-RISE") -> (w2701:string[])
                            n1432 = Build Array(w2699) -> (w2700:dbl[])
                            n1433 = TDMS Write(0:w2697, 5:"TEST PASS", 7:w2701, 9:w2700) -> (15:w2703:errorcluster)  [unwired: 2 in, 3 out]
                            n1434 = local write "data file error"(w2703) -> ()
                          }
                          frame #1 {
                            n1435 = Bundle(cluster=w2704, "STATUS"="T-RISE PASS") -> (w2706:T4)  [unwired: 2 in]
                            n1436 = local write "RESULT LAB03-1"(TRUE) -> ()
                            n1437 = local write "DISP LAB03-1"(w2706) -> ()
                          }
                        }
                      }
                      frame False {
                      }
                    }
                  }
                }
              }
              frame #5 {
                # "LAB03-2"
                n1438 = Equal?(x=w2709, y=2) -> (x = y?=w2712:bool)
                n1439 = local read "DISP LAB03-2"() -> (w2714:T4)
                n1440 = Unbundle(w2714) -> ("STATUS"=w2715:string)  [unwired: 2 out]
                n1441 = Equal?(x=w2715, y="RUN") -> (x = y?=w2711:bool)
                n1442 = And(x=w2711, y=w2712) -> (x .and. y?=w2710:bool)
                n1443 = case shown="True" w2710 {
                  tunnel: w2714 -> [_ w2718]
                  tunnel: w2708 -> [_ w2721]
                  frame False {
                  }
                  frame True {
                    n1444 = local read "SET LAB03-2"() -> (w2720:T5)
                    n1445 = local read "TDMS LAB03-2"() -> (w2717:refnum<k34>)
                    n1446 = Unbundle(w2718) -> ("CYCLE"=w2722:dbl)  [unwired: 2 out]
                    n1447 = Unbundle(w2720) -> ("T-RISE mins"=w2719:dbl)  [unwired: 4 out]
                    n1448 = Greater Or Equal?(x=w2722, y=w2721) -> (x >= y?=w2723:bool)
                    n1449 = case shown="True" w2723 {
                      tunnel: w2719 -> [w2726 _]
                      tunnel: w2718 -> [w2725 _]
                      tunnel: w2717 -> [w2724 _]
                      frame True {
                        n1450 = stacked-sequence {
                          tunnel: w2726 -> [w2729 _]
                          tunnel: w2725 -> [_ w2734]
                          tunnel: w2724 -> [w2727 _]
                          frame #0 {
                            n1451 = Build Array("T-RISE") -> (w2731:string[])
                            n1452 = Build Array(w2729) -> (w2730:dbl[])
                            n1453 = TDMS Write(0:w2727, 5:"TEST PASS", 7:w2731, 9:w2730) -> (15:w2733:errorcluster)  [unwired: 2 in, 3 out]
                            n1454 = local write "data file error"(w2733) -> ()
                          }
                          frame #1 {
                            n1455 = Bundle(cluster=w2734, "STATUS"="T-RISE PASS") -> (w2736:T4)  [unwired: 2 in]
                            n1456 = local write "RESULT LAB03-2"(TRUE) -> ()
                            n1457 = local write "DISP LAB03-2"(w2736) -> ()
                          }
                        }
                      }
                      frame False {
                      }
                    }
                  }
                }
              }
              frame #6 {
                # "LAB04-1"
                n1458 = Equal?(x=w2739, y=2) -> (x = y?=w2742:bool)
                n1459 = local read "DISP LAB04-1"() -> (w2744:T4)
                n1460 = Unbundle(w2744) -> ("STATUS"=w2745:string)  [unwired: 2 out]
                n1461 = Equal?(x=w2745, y="RUN") -> (x = y?=w2741:bool)
                n1462 = And(x=w2741, y=w2742) -> (x .and. y?=w2740:bool)
                n1463 = case shown="True" w2740 {
                  tunnel: w2744 -> [_ w2748]
                  tunnel: w2738 -> [_ w2751]
                  frame False {
                  }
                  frame True {
                    n1464 = local read "SET LAB04-1"() -> (w2750:T5)
                    n1465 = local read "TDMS LAB04-1"() -> (w2747:refnum<k34>)
                    n1466 = Unbundle(w2748) -> ("CYCLE"=w2752:dbl)  [unwired: 2 out]
                    n1467 = Unbundle(w2750) -> ("T-RISE mins"=w2749:dbl)  [unwired: 4 out]
                    n1468 = Greater Or Equal?(x=w2752, y=w2751) -> (x >= y?=w2753:bool)
                    n1469 = case shown="True" w2753 {
                      tunnel: w2749 -> [w2756 _]
                      tunnel: w2748 -> [w2755 _]
                      tunnel: w2747 -> [w2754 _]
                      frame True {
                        n1470 = stacked-sequence {
                          tunnel: w2756 -> [w2759 _]
                          tunnel: w2755 -> [_ w2764]
                          tunnel: w2754 -> [w2757 _]
                          frame #0 {
                            n1471 = Build Array("T-RISE") -> (w2761:string[])
                            n1472 = Build Array(w2759) -> (w2760:dbl[])
                            n1473 = TDMS Write(0:w2757, 5:"TEST PASS", 7:w2761, 9:w2760) -> (15:w2763:errorcluster)  [unwired: 2 in, 3 out]
                            n1474 = local write "data file error"(w2763) -> ()
                          }
                          frame #1 {
                            n1475 = Bundle(cluster=w2764, "STATUS"="T-RISE PASS") -> (w2766:T4)  [unwired: 2 in]
